vi "cmc-inclass-coordinates.vi"(8 "error in (no error)":errorcluster, 10 "Angle(radians)":dbl, 11 "Radius":dbl) -> (0 "error out":errorcluster, 2 "y coordinate":dbl, 3 "x coordinate":dbl)   [LabVIEW 2010]
doc: "This VI converts the cylindrical polar coordinates to cartesian coordinates. NOTE: Input angle is available in radians only and the input radius is in the same units as x & y.\n\nCreated by Clair Cunningham\nRIT - Mechanical Engineering\nFall Quarter 2011"
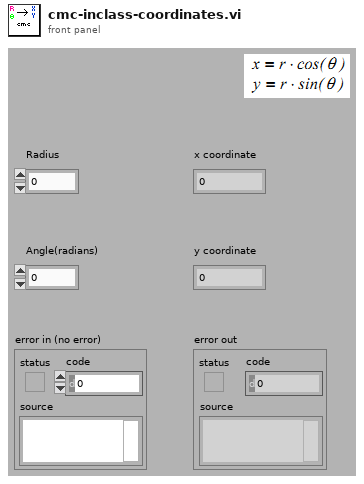
[diagram p1: front panel]
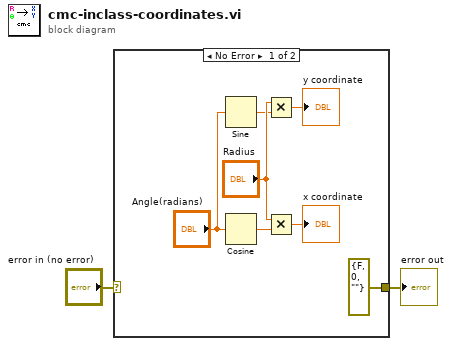
[diagram p0: block diagram]
diagram:
  n1 = case shown="No Error" "error in (no error)" {
    selector: "error in (no error)" -> [_ w10]
    tunnel: [errorcluster {"status"=FALSE, "code"=0, "source"=""} ("error IO") w10] -> w1
    frame No Error {
      n2 = Sine(x="Angle(radians)") -> (sin(x)=w6:dbl)
      n3 = Cosine(x="Angle(radians)") -> (cos(x)=w7:dbl)
      n4 = Multiply(x="Radius", y=w6) -> (x*y=→"y coordinate":dbl)
      n5 = Multiply(x="Radius", y=w7) -> (x*y=→"x coordinate":dbl)
    }
    frame Error {
    }
  }
  "error out" <- w1
